vi "Add the Current DateTime.vi"(11 "string":string) -> (3 "concatenated string":string)   [LabVIEW 2021]
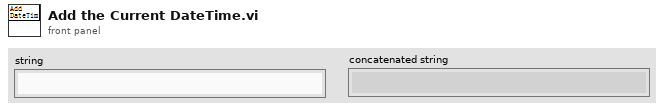
[diagram p1: front panel]
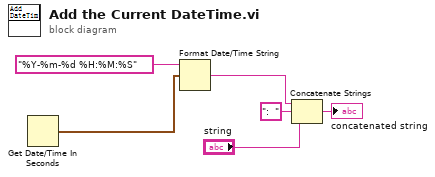
[diagram p0: block diagram]
diagram:
  n1 = Get Date/Time In Seconds() -> (seconds since 1Jan1904=w5:timestamp)
  n2 = Format Date/Time String(time format string (%c)="%Y-%m-%d %H:%M:%S", seconds (now)=w5) -> (date/time string=w4:string)  [unwired: 1 in]
  n3 = Concatenate Strings(w4, ":  " ("string"), "string") -> (→"concatenated string":string)
